vi "PlotSingleRSOHcube.vi"() -> ()   [LabVIEW 2014]
uses:
  TypeDefs/RectHatch.ctl
  TypeDefs/PowerSpeed.ctl
panel:
  in  "OHpows":dbl[](array[numeric])=[50.0, 75.0, 100.0, 125.0, 250.0]
  in  "EndLayer":u32=170
  in  "Display":T1={"Mode"=enum."Inherit Value", "PointSize"=1.0, "LineWidth"=1.0}
  in  "HighPower":dbl=500.0
  in  "StartLayer":u32=170
  in  "HatchPow":T2={"Power"=300.0, "Mark Speed"=400.0, "Jump Speed"=1000.0}
  in  "RectHatch":T3={"Width"=10.0, "Height"=10.0, "Angle"=45.0, "OffX"=0.1, "OffY"=0.1, "Spacing"=0.1, "IslandSize"=0.1} {"IslandSize" format="%#_13g"; "Spacing" format="%#_13g"; "OffY" format="%#_13g"; "OffX" format="%#_13g"; "Height" format="%#_13g"; "Width" format="%#_13g"}
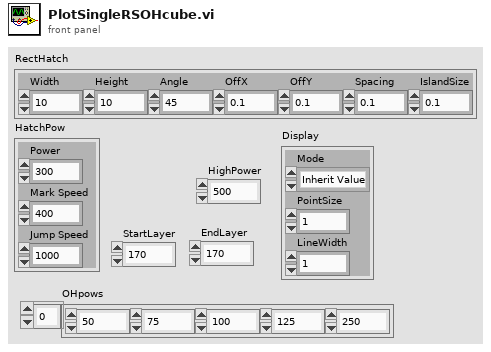
[diagram p1: front panel]
types:
  T1 = cluster{"Mode":enum16{"Inherit Value", "Points", "Wireframe", "Polygons"}, "PointSize":sgl, "LineWidth":sgl}
  T2 = typedef "PowerSpeed.ctl" = cluster{"Power":dbl, "Mark Speed":dbl, "Jump Speed":dbl}
  T3 = typedef "RectHatch.ctl" = cluster{"Width":dbl, "Height":dbl, "Angle":sgl, "OffX":dbl, "OffY":dbl, "Spacing":dbl, "IslandSize":dbl}
  T4 = typedef "PathSupreme.ctl" = cluster{"VelocityProfiles":T5[], "Path":T6}
  T5 = typedef "VelocityProfile.ctl" = cluster{"ID":u32, "Velocity":dbl, "Mode":string, "tV1":u32, "tV2":u32, "tL1":u32, "tL2":u32}
  T6 = typedef "PathCut.ctl" = cluster{"Type":string, "Tag":string, "Segments":T7[]}
  T7 = typedef "Segment.ctl" = cluster{"SegmentID":u16, "Power":sgl, "idxVelocityProfile":u16, "End":cluster{"X":sgl, "Y":sgl}}
  T8 = typedef "Point3D.ctl" = cluster{"X":sgl, "Y":sgl, "Z":sgl}
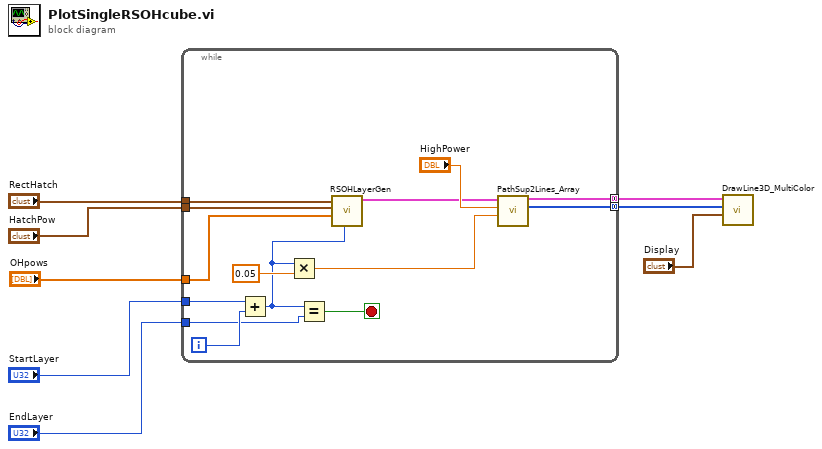
[diagram p0: block diagram]
diagram:
  n1 = while {
    tunnel: [w22] -> w8 mode=concatenating
    tunnel: [w21] -> w7 mode=concatenating
    tunnel: "RectHatch" -> [w20]
    tunnel: "HatchPow" -> [w19]
    tunnel: "StartLayer" -> [w15]
    tunnel: "EndLayer" -> [w13]
    tunnel: "OHpows" -> [w9]
    i -> [w14]
    stop <- w16 stop-if-true
    n2 = Add(x=w15, y=w14) -> (x+y=w12:u32)
    n3 = Multiply(x=w12, y=0.05) -> (x*y=w11:dbl)
    n4 = Equal?(x=w12, y=w13) -> (x = y?=w16:bool)
    n5 = call "RSOHLayerGen.vi"("Layer"=w12, "OHpows"=w9, "HatchPow"=w19, "RectHatch"=w20) -> ("PathSups"=w10:T4[])  [unwired: 5 in, 2 out]
    n6 = call "PathSup2Lines_Array.vi"("Z"=w11, "HighPower"="HighPower", "PathSupIn"=w10) -> ("Colors"=w21:u32[], "Lines"=w22:cluster{"P0":T8, "P1":T8}[])  [unwired: 7 in]
  }
  n7 = call "DrawLine3D_MultiColor.vi"("Display"="Display", "Colors"=w7, "Lines"=w8) -> ()  [unwired: 9 in]
